vi "ep_Highpass IIR Filter Design.vi"(8 "error in (no error)":errorcluster, 11 "fs":dbl) -> (0 "error out":errorcluster, 3 "highpass IIR Filter":T1 {"Forward Coefficients" format="%.4f"; "Reverse Coefficients" format="%.4f"})   [LabVIEW 2014, in "NI_EP_Motor Monitoring.lvlib"]
uses:
  <vilib>/addons/Electrical Power/Motor Monitoring/NI_EP_Motor Monitoring.lvlib
  <vilib>/Analysis/3filter.llb/Filter Passband Type.ctl
  <vilib>/Analysis/3filter.llb/Filter Frequence Specification (Design).ctl
  <vilib>/Analysis/3filter.llb/Filter Ripple Specification (Design).ctl
  <vilib>/Analysis/NI_AALBase.lvlib
  <vilib>/Analysis/NI_AAL_Filter.lvlib
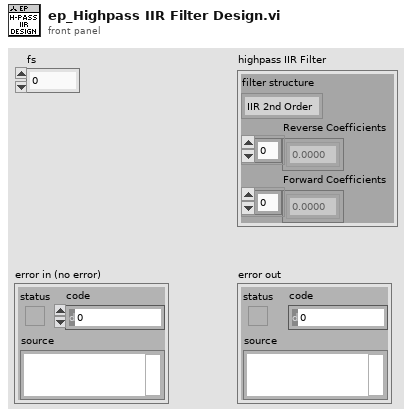
[diagram p1: front panel]
types:
  T1 = cluster{"filter structure":enum32{"IIR 2nd Order", "IIR 4th Order"}, "Reverse Coefficients":dbl[], "Forward Coefficients":dbl[]}
  T2 = typedef "NI_AAL_Filter.lvlib/Filter Ripple Specification (Design).ctl" = cluster{"passband":dbl, "stopband":dbl, "dB/linear? (T: dB)":bool}
  T3 = typedef "NI_AAL_Filter.lvlib/Filter Frequence Specification (Design).ctl" = cluster{"lower pass freq":dbl, "lower stop freq":dbl, "higher pass freq":dbl, "higher stop freq":dbl}
  T4 = typedef "NI_AALBase.lvlib/Filter Passband Type.ctl" = enum32{"Lowpass", "Highpass", "Bandpass", "Bandstop"}
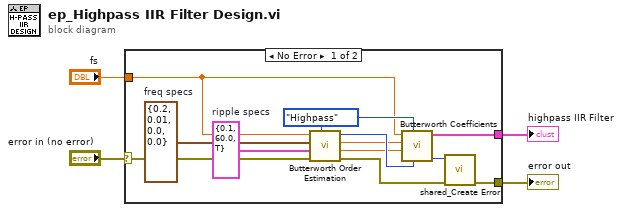
[diagram p0: block diagram]
diagram:
  n1 = case shown="No Error" "error in (no error)" {
    selector: "error in (no error)" -> [w12 w17]
    tunnel: [w7 w17] -> w3
    tunnel: "fs" -> [w5 _]
    tunnel: [w6 _] -> w1
    frame No Error {
      w10 = T2 {"passband"=0.1, "stopband"=60.0, "dB/linear? (T: dB)"=TRUE}  # ripple specs
      w11 = T3 {"lower pass freq"=0.2, "lower stop freq"=0.01, "higher pass freq"=0.0, "higher stop freq"=0.0}  # freq specs
      w13 = Filter_Passband_Type."Highpass" ("filter type")
      n2 = call <vilib>:"Butterworth Order Estimation.vi"("filter type"=w13, "error in (no error)"=w12, "ripple specs"=w10, "freq specs"=w11, "sampling freq: fs"=w5) -> ("error out"=w8:errorcluster, "low cutoff freq"=w14:dbl, "high cutoff freq"=w15:dbl, "estimated order"=w16:i32)  [unwired: 3 in]
      n3 = call <vilib>:"Butterworth Coefficients.vi"("order"=w16, "filter type"=w13, "low cutoff freq: fl"=w14, "high cutoff freq: fh"=w15, "sampling freq: fs"=w5) -> ("error"=w9:i32, "IIR Filter Cluster"=w6:T1)  [unwired: 5 in]
      n4 = call <vilib>:"shared_Create Error.vi"("error in (no error)"=w8, "error code (0)"=w9) -> ("error out"=w7:errorcluster)  [unwired: 9 in]
    }
    frame Error {
    }
  }
  "error out" <- w3
  "highpass IIR Filter" <- w1
